vi "Add Part.vi"(8 "error in":errorcluster, 10 "PartType":i32(ring) items=["SharedString", "Worksheet", "WorkbookStyles"], 11 "SpreadsheetDoc in":refnum<k24>) -> (0 "error out":errorcluster, 2 "OpenXmlPart":refnum<k24>, 3 "SpreadsheetDoc out":refnum<k24>)   [LabVIEW 2021, in "Open Xml.lvlib"]
uses:
  Open Xml.lvlib
  D:/git/Open-Xml-LabVIEW/dll/DocumentFormat.OpenXml.dll
  dll/DocumentFormat.OpenXml.dll
  D:/git/Open-Xml-LabVIEW/dll/DocumentFormat.OpenXml.Framework.dll
  dll/DocumentFormat.OpenXml.Framework.dll
  D:/git/Open-Xml-LabVIEW/dll/OpenXmlGenericsWrapper.dll
  dll/OpenXmlGenericsWrapper.dll
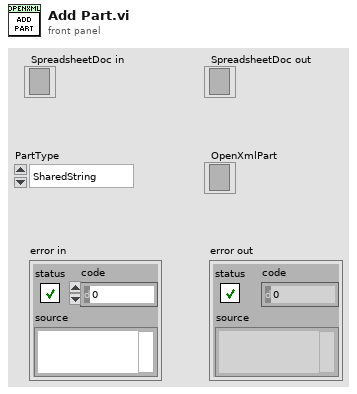
[diagram p1: front panel]
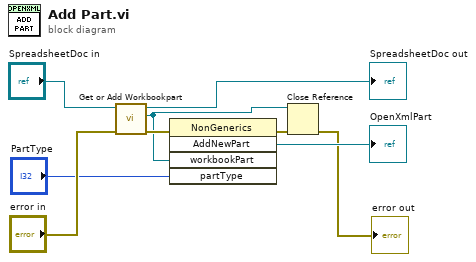
[diagram p0: block diagram]
diagram:
  n1 = call "Get or Add Workbookpart.vi"("error in"="error in", "SpreadsheetDoc in"="SpreadsheetDoc in") -> ("error out"=w8:errorcluster, "WorkbookPart"=w1:refnum<k24>, "SpreadsheetDoc out"=→"SpreadsheetDoc out":refnum<k24>)  [unwired: 7 in]
  n2 = invoke class="NonGenerics" method="AddNewPart"(error in=w8, "workbookPart"=w1, "partType"="PartType") -> (error out=w5:errorcluster, "AddNewPart"=→"OpenXmlPart":refnum<k24>)  [unwired: 2 in, 3 out]
  n3 = Close Reference(reference=w1, error in (no error)=w5) -> (error out=→"error out":errorcluster)
